vi "ReadAI_Info.vi"(0 "reference in":refnum<class "DAQ_Base.lvclass">, 5 "error in (no error)":errorcluster) -> (10 "采集通道名称":string[](array[string]), 12 "DAQSettings":T1={"SampleSettings"={"samples per channel"=100, "SampleRate"=1000.0, "TansMaxLength"=500000.0, "ReadTimeOut"=10.0, "时钟源"=""}, "AI_ChannelSettings"={"AI_SettingsArry"=[]}, "AO_ChannelSettings"={"布尔"=FALSE}, "Cnt_ChannelSettings"={"Cnt_ChannelSettings"=[]}} {"Cnt_ChannelSettings"."Cnt_ChannelSettings"."decoding type" items=["X1"=10090, "X2"=10091, "X4"=10092, "双脉冲计数"=10313]; "Cnt_ChannelSettings"."Cnt_ChannelSettings"."z index phase" items=["A High B High"=10040, "A High B Low"=10041, "A Low B High"=10042, "A Low B Low"=10043, ""=0]; "Cnt_ChannelSettings"."Cnt_ChannelSettings"."单位" items=["Radians"=10273, "Degrees"=10146, "Meters"=10219, "Inches"=10379, "Ticks"=10304, "From Custom Scale"=10065]; "AI_ChannelSettings"."AI_SettingsArry"."标定系数"."Offset" format="%_4g"; "AI_ChannelSettings"."AI_SettingsArry"."标定系数"."Scale" format="%.4g"; "AI_ChannelSettings"."AI_SettingsArry"."shunt resistor location" items=["默认"=-1, "内部"=10200, "外部"=10167]; "AI_ChannelSettings"."AI_SettingsArry"."external shunt resistor value" format="%0.2f"; "AI_ChannelSettings"."AI_SettingsArry"."输入信号类型" items=["默认"=-1, "RSE"=10083, "NRSE"=10078, "差分"=10106, "伪差分"=12529]; "AI_ChannelSettings"."AI_SettingsArry"."单位" items=["安培"=10342, "伏特"=10348, "来自自定义换算"=10065]}, 14 "reference out":refnum<class "DAQ_Base.lvclass">, 15 "模拟量名称":string[](array[string]), 16 "模拟量数量":i32, 17 "标定系数Arry":cluster{"Scale":dbl, "Offset":dbl}[](array[cluster]), 18 "AI_ChannelSettings":T3 {"AI_SettingsArry"."标定系数"."Offset" format="%_4g"; "AI_SettingsArry"."标定系数"."Scale" format="%.4g"; "AI_SettingsArry"."shunt resistor location" items=["默认"=-1, "内部"=10200, "外部"=10167]; "AI_SettingsArry"."external shunt resistor value" format="%0.2f"; "AI_SettingsArry"."输入信号类型" items=["默认"=-1, "RSE"=10083, "NRSE"=10078, "差分"=10106, "伪差分"=12529]; "AI_SettingsArry"."单位" items=["安培"=10342, "伏特"=10348, "来自自定义换算"=10065]}, 19 "error out":errorcluster)   [LabVIEW 2020, in "DAQ.lvlib" / "DAQ_Base.lvclass"]
uses:
  DAQ_Base.lvclass
  protected/AI_ChannelSettings.ctl
  protected/DAQSettings.ctl
  protected/SampleSettings.ctl
  protected/AO_ChannelSettings.ctl
  protected/Cnt_ChannelSettings.ctl
panel:
  out "模拟量物理值名称":string[](array[string])
  out "CntName":string[](array[string])
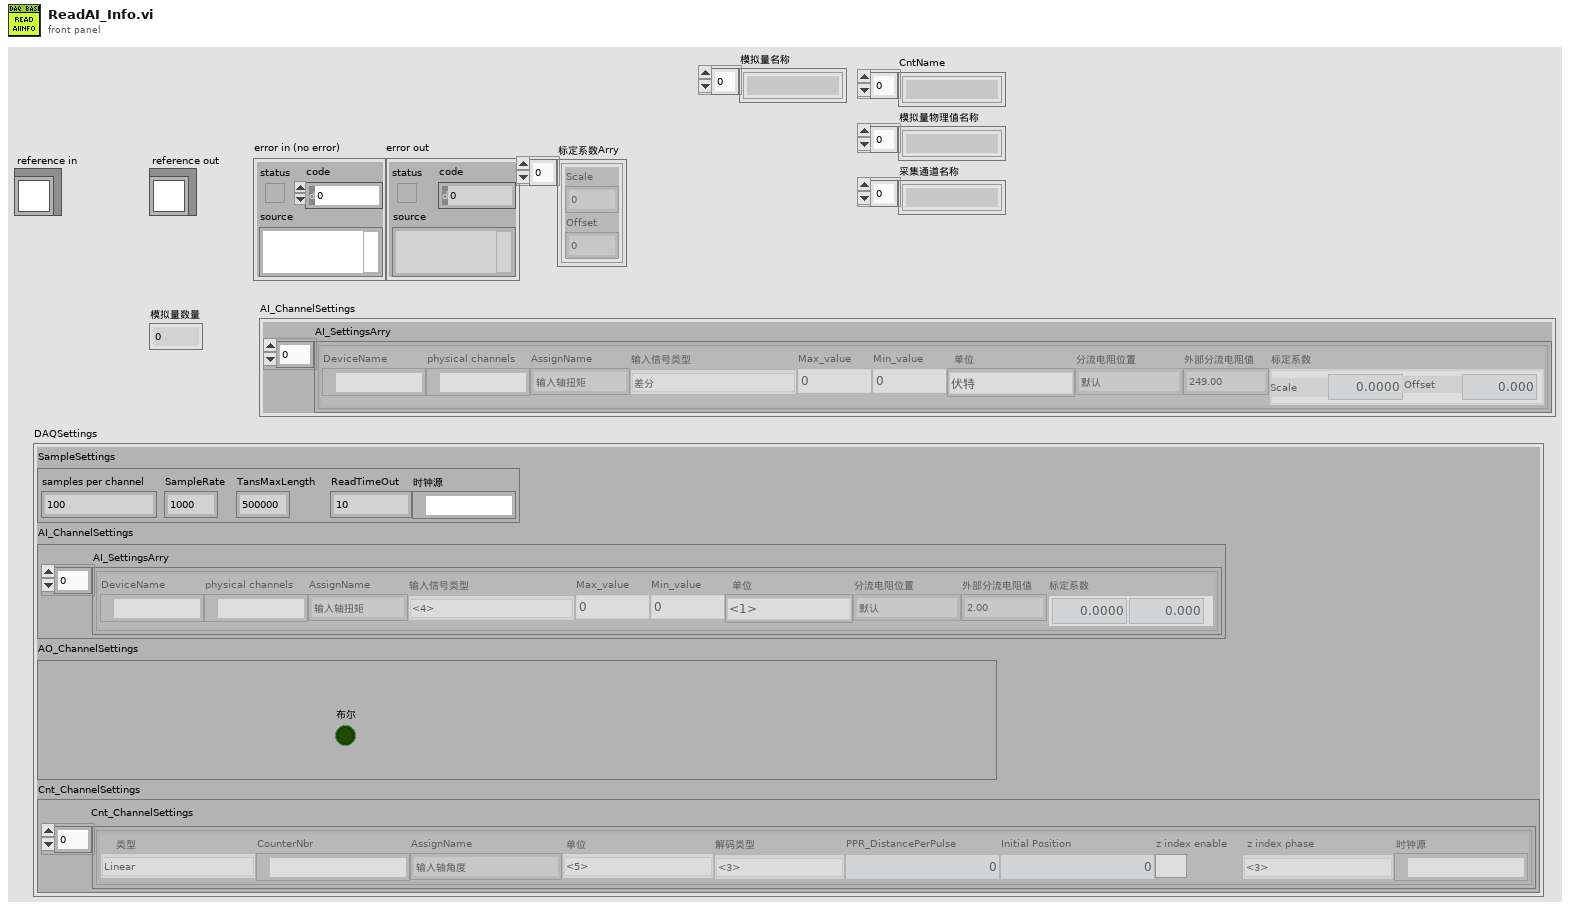
[diagram p1: front panel]
types:
  T1 = typedef "DAQ.lvlib/DAQ_Base.lvclass/DAQSettings.ctl" = cluster{"SampleSettings":T2, "AI_ChannelSettings":T3, "AO_ChannelSettings":T5, "Cnt_ChannelSettings":T6}
  T2 = typedef "DAQ.lvlib/DAQ_Base.lvclass/SampleSettings.ctl" = cluster{"samples per channel":i32, "SampleRate":dbl, "TansMaxLength":dbl, "ReadTimeOut":dbl, "时钟源":tag}
  T3 = typedef "DAQ.lvlib/DAQ_Base.lvclass/AI_ChannelSettings.ctl" = cluster{"AI_SettingsArry":cluster{"DeviceName":tag, "physical channels":tag, "AssignName":string, "输入信号类型":T4, "Max_value":dbl, "Min_value":dbl, "单位":i32, "shunt resistor location":i32, "external shunt resistor value":dbl, "标定系数":cluster{"Scale":dbl, "Offset":dbl}}[]}
  T4 = typedef "AI信号类型.ctl" = i32
  T5 = typedef "DAQ.lvlib/DAQ_Base.lvclass/AO_ChannelSettings.ctl" = cluster{"布尔":bool}
  T6 = typedef "DAQ.lvlib/DAQ_Base.lvclass/Cnt_ChannelSettings.ctl" = cluster{"Cnt_ChannelSettings":cluster{"类型":enum16{"Linear", "Rotate"}, "CounterNbr":tag, "AssignName":string, "单位":u16, "decoding type":u16, "PPR_DistancePerPulse":dbl, "Initial Position ":dbl, "z index enable":bool, "z index phase":i32, "source":tag}[]}
  T7 = cluster{"DeviceName":tag, "physical channels":tag, "AssignName":string, "输入信号类型":T4, "Max_value":dbl, "Min_value":dbl, "单位":i32, "shunt resistor location":i32, "external shunt resistor value":dbl, "标定系数":cluster{"Scale":dbl, "Offset":dbl}}[]
  T8 = cluster{"类型":enum16{"Linear", "Rotate"}, "CounterNbr":tag, "AssignName":string, "单位":u16, "decoding type":u16, "PPR_DistancePerPulse":dbl, "Initial Position ":dbl, "z index enable":bool, "z index phase":i32, "source":tag}[]
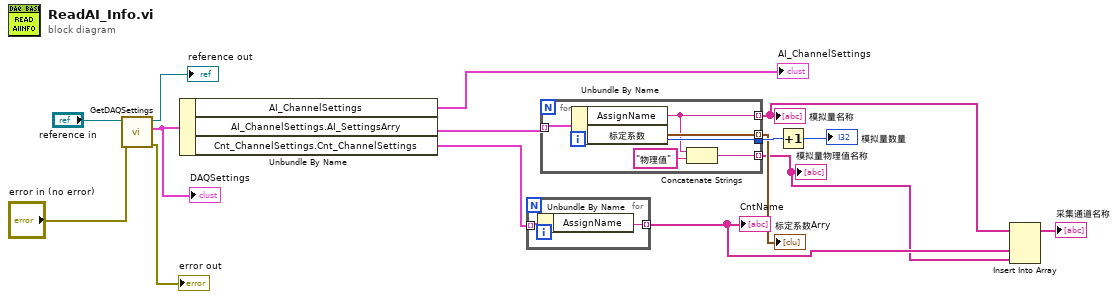
[diagram p0: block diagram]
diagram:
  n1 = call-dynamic "GetDAQSettings.vi"("error in (no error)"="error in (no error)", "reference in"="reference in") -> ("error out"=→"error out":errorcluster, "DAQSettings"=w15:T1, "reference out"=→"reference out":refnum<class "DAQ_Base.lvclass">)  [unwired: 7 in]
  "DAQSettings" <- w15
  n2 = Unbundle By Name(w15) -> ("AI_ChannelSettings"=→"AI_ChannelSettings":T3, "AI_ChannelSettings.AI_SettingsArry"=w14:T7, "Cnt_ChannelSettings.Cnt_ChannelSettings"=w5:T8)
  n3 = for {
    tunnel: w5 -> [w17] mode=indexing
    tunnel: [w16] -> w2 mode=indexing
    n4 = Unbundle By Name(w17) -> ("AssignName"=w16:string)
  }
  "CntName" <- w2
  n5 = for {
    tunnel: w14 -> [w23] mode=indexing
    tunnel: [w20] -> w3 mode=indexing
    tunnel: [w22] -> w13
    tunnel: [w21] -> w7 mode=indexing
    tunnel: [w18] -> w1 mode=indexing
    i -> [w22]
    n6 = Unbundle By Name(w23) -> ("AssignName"=w20:string, "标定系数"=w21:cluster{"Scale":dbl, "Offset":dbl})
    n7 = Concatenate Strings(w20, "物理值" ("字符串")) -> (w18:string)
  }
  "模拟量名称" <- w3
  "标定系数Arry" <- w7
  "模拟量物理值名称" <- w1
  n8 = Increment(x=w13) -> (x+1=→"模拟量数量":i32)
  n9 = Insert Into Array(array=w3, new element #1=w2, new element #2=w1) -> (→"采集通道名称":string[])  [unwired: 1 in]
